vi "Write Resource Data ref.vi"(8 "error in (no error)":errorcluster, 10 "Resource Data ref":refnum<data-value>, 11 "VI Data in":refnum<class "VI Data.lvclass">) -> (0 "error out":errorcluster, 3 "VI Data out":refnum<class "VI Data.lvclass">)   [LabVIEW 2013, in "SET Project Data.lvlib" / "VI Data.lvclass"]
uses:
  VI Data.lvclass
  Resource Data Class/Resource Data.lvclass
  VI Data.lvclass/VI Data.ctl
  Control Classes/GObject/GObject.lvclass/GObject.ctl
  Control Classes/GObject/GObject.lvclass
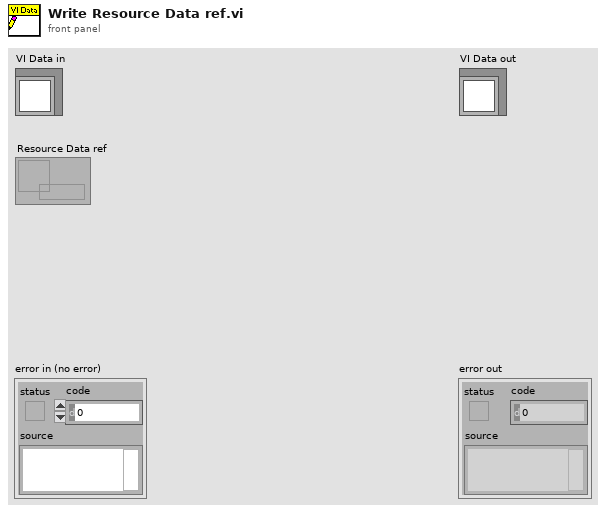
[diagram p1: front panel]
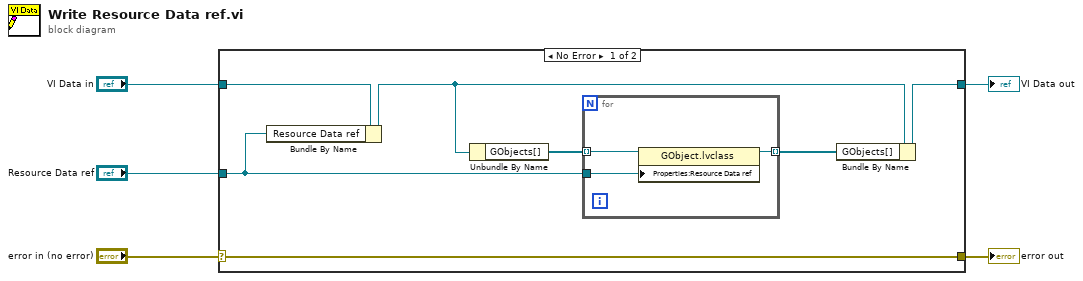
[diagram p0: block diagram]
diagram:
  n1 = case shown="No Error" "error in (no error)" {
    selector: "error in (no error)" -> [w12 w16]
    tunnel: [w12 w16] -> w4
    tunnel: [w7 w17] -> w2
    tunnel: "VI Data in" -> [w11 w17]
    tunnel: "Resource Data ref" -> [w9 _]
    frame No Error {
      n2 = Bundle By Name(cluster=w11, "Resource Data ref"=w9) -> (w8:refnum<class "VI Data.lvclass">)
      n3 = Unbundle By Name(w8) -> ("GObjects[]"=w10:refnum<class "GObject.lvclass">[])
      n4 = for {
        tunnel: w10 -> [w15] mode=indexing
        tunnel: w9 -> [w14]
        tunnel: [w13] -> w6 mode=indexing
        n5 = property class="GObject.lvclass"(reference=w15, "Properties:Resource Data ref"=w14) -> (reference out=w13:refnum<class "GObject.lvclass">)  [unwired: 1 in, 1 out]
      }
      n6 = Bundle By Name(cluster=w8, "GObjects[]"=w6) -> (w7:refnum<class "VI Data.lvclass">)
    }
    frame Error {
    }
  }
  "error out" <- w4
  "VI Data out" <- w2
